vi "AutoGrabCamera.vi"(8 "error in":errorcluster) -> (0 "error out":errorcluster, 3 "Session Out Array":T1[](array[typedef]))   [LabVIEW 2015]
uses:
  <vilib>/userdefined/High Color/IMAQdx.ctl
  <vilib>/vision/driver/NI_Vision_Acquisition_Software.lvlib
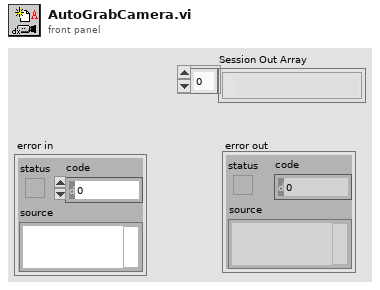
[diagram p1: front panel]
types:
  T1 = typedef "IMAQdx.ctl" = refnum<k21>
  T2 = cluster{"Type":u32, "Version":u32, "Flags":u32, "SerialNumberHigh":u32, "SerialNumberLow":u32, "BusType":u32, "InterfaceName":string, "VendorName":string, "ModelName":string, "CameraFileName":string, "CameraAttributeURL":string}[]
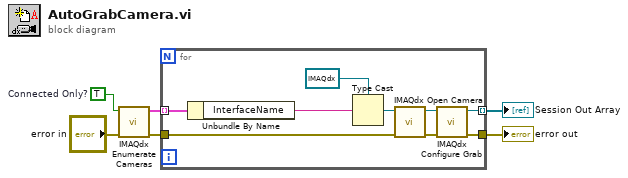
[diagram p0: block diagram]
diagram:
  w5 = TRUE  # Connected Only?
  n1 = call <vilib>:"IMAQdx Enumerate Cameras.vi"("error in"="error in", "Connected Only? (Yes)"=w5) -> ("error out"=w3:errorcluster, "Camera Information Array"=w6:T2)  [unwired: 8 out]
  n2 = for {
    tunnel: w6 -> [w15] mode=indexing
    tunnel: w3 -> [w9]
    tunnel: [w8] -> w2 mode=indexing
    tunnel: [w7] -> w1
    n3 = Unbundle By Name(w15) -> ("InterfaceName"=w13:string)
    n4 = Type Cast(type=T1 refnum ("Session In"), x=w13) -> (*(type *) &x=w12:T1)
    n5 = call <vilib>:"IMAQdx Open Camera.vi"("error in"=w9, "Session In"=w12) -> ("error out"=w10:errorcluster, "Session Out"=w11:T1)  [unwired: 1 in, 7 out]
    n6 = call <vilib>:"IMAQdx Configure Grab.vi"("error in"=w10, "Session In"=w11) -> ("error out"=w7:errorcluster, "Session Out"=w8:T1)  [unwired: 8 out]
  }
  "error out" <- w1
  "Session Out Array" <- w2
